vi "Scale Window.vi"(0 "VI in":refnum<vi>, 11 "error in (no error)":errorcluster) -> (4 "VI out":refnum<vi>, 15 "error out":errorcluster)   [LabVIEW 2016, in "LV Doc.lvclass"]
uses:
  LV Doc.lvclass
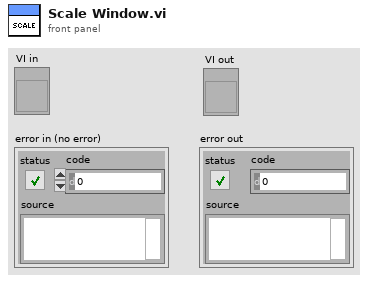
[diagram p1: front panel]
types:
  T1 = enum16{"No Scaling", "Scale All Objects", "Scale Single Object"}
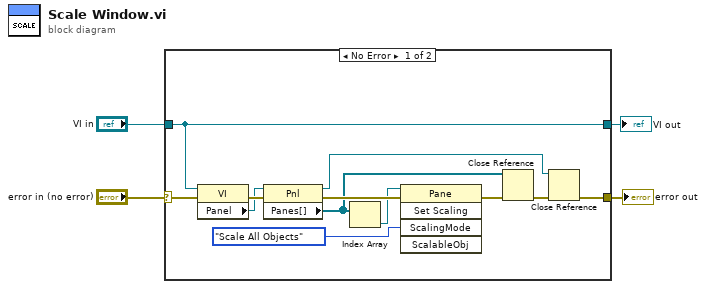
[diagram p0: block diagram]
diagram:
  n1 = case shown="No Error" "error in (no error)" {
    selector: "error in (no error)" -> [w15 w18]
    tunnel: [w6 w18] -> w4
    tunnel: "VI in" -> [w9 w17]
    tunnel: [w9 w17] -> w1
    frame No Error {
      n2 = property class="VI"(reference=w9, error in=w15) -> (error out=w13:errorcluster, "Panel"=w10:refnum<vi>)  [unwired: 1 out]
      n3 = property class="Pnl"(reference=w10, error in=w13) -> (reference out=w5:refnum<vi>, error out=w14:errorcluster, "Panes[]"=w8:refnum<vi>[])
      n4 = Index Array(array=w8) -> (element=w11:refnum<vi>)  [unwired: 1 in]
      n5 = invoke class="Pane" method="Set Scaling"(reference=w11, error in=w14, "ScalingMode"=T1."Scale All Objects" ("Scaling Mode")) -> (error out=w16:errorcluster)  [unwired: 2 in, 4 out]
      n6 = Close Reference(reference=w8, error in (no error)=w16) -> (error out=w7:errorcluster)
      n7 = Close Reference(reference=w5, error in (no error)=w7) -> (error out=w6:errorcluster)
    }
    frame Error {
    }
  }
  "error out" <- w4
  "VI out" <- w1
